vi "List Sensors.vi"(8 "error in (no error)":errorcluster, 11 "Create Test Channel Model in":refnum<class "Create Test Channel Model.lvclass">) -> (0 "error out":errorcluster, 3 "Create Test Channel Model out":refnum<class "Create Test Channel Model.lvclass">)   [LabVIEW 2013, in "Create Test Channel Model.lvlib" / "Create Test Channel Model.lvclass"]
uses:
  Create Test Channel Model.lvclass
  Create Test Channel Model.lvclass/Create Test Channel Model.ctl
  Common/File IO/File IO.lvlib
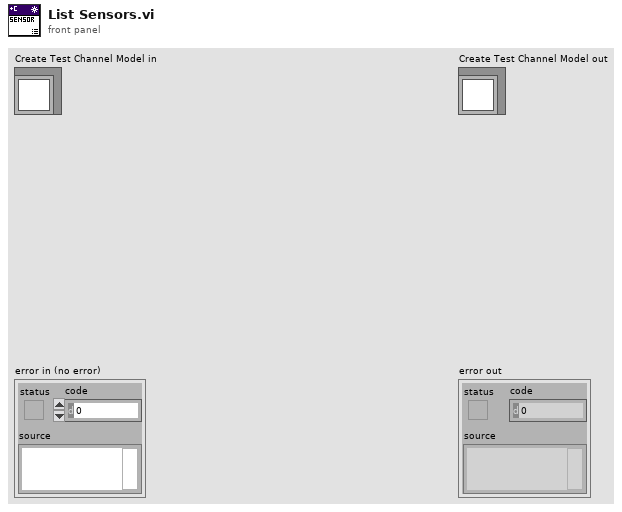
[diagram p1: front panel]
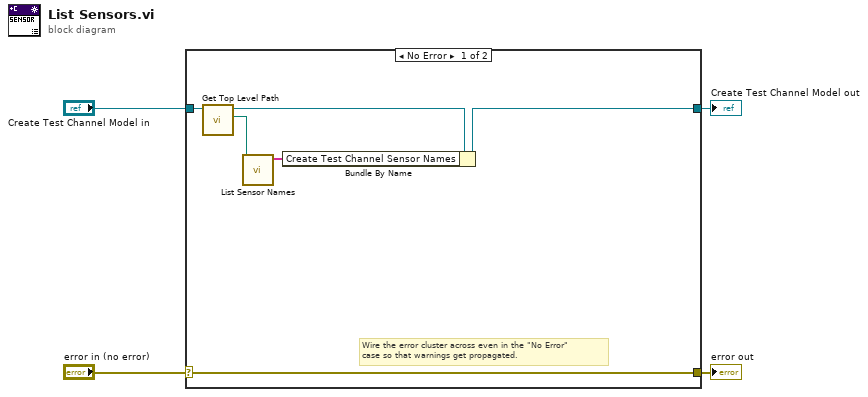
[diagram p0: block diagram]
diagram:
  n1 = case shown="No Error" "error in (no error)" {
    selector: "error in (no error)" -> [w9 w12]
    tunnel: [w9 w12] -> w3
    tunnel: [w7 w11] -> w1
    tunnel: "Create Test Channel Model in" -> [w10 w11]
    frame No Error {
      # "Wire the error cluster across even in the \"No Error\"\ncase so that warnings get propagated."
      n2 = call-dynamic "Get Top Level Path.vi"("Abstract Model in"=w10) -> ("Top Level Path"=w5:path, "Abstract Model out"=w8:refnum<class "Create Test Channel Model.lvclass">)  [unwired: 8 in, 1 out]
      n3 = call "List Sensor Names.vi"("Top Level Path"=w5) -> ("Sensor Names"=w6:string[])  [unwired: 10 in]
      n4 = Bundle By Name(cluster=w8, "Create Test Channel Sensor Names"=w6) -> (w7:refnum<class "Create Test Channel Model.lvclass">)
    }
    frame Error {
    }
  }
  "error out" <- w3
  "Create Test Channel Model out" <- w1
